vi "LI-U8 convert hex string to U8 array number .vi"(4 "hex string (MSD 1st)":string) -> (1 "Large number -U8":T1)   [LabVIEW 2013]
doc: "Converts a hex string (with MSD first) to large integer in U8 array format."
uses:
  User Access Type defs/Large number - U8 array.ctl
panel:
  # "<<LSD"
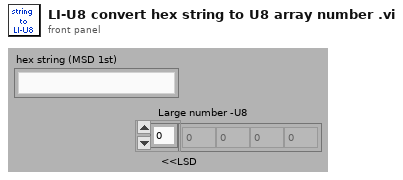
[diagram p1: front panel]
types:
  T1 = typedef "Large number - U8 array.ctl" = u8[]
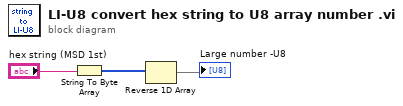
[diagram p0: block diagram]
diagram:
  n1 = String To Byte Array(string="hex string (MSD 1st)") -> (unsigned byte array=w2:u8[])
  n2 = Reverse 1D Array(array=w2) -> (reversed array=→"Large number -U8":u8[])
